vi "f_10_DiDtOff.vi"(0 "file path (IN)":path, 1 "Project #":string, 2 "Request #":string, 3 "TEST #":string, 5 "error in (no error)":errorcluster, 6 "ICE":dbl) -> (11 "Di (A)":dbl, 13 "Dt (ns)":dbl, 14 "file path (OUT)":path, 15 "Di/Dt (A/us)":dbl, 16 "DONE Di/Dt OFF":bool, 19 "error out":errorcluster)   [LabVIEW 2020]
uses:
  GlobIndSw1.vi
  <vilib>/Waveform/WDTOps.llb/WDT Waveform Duration DBL.vi
  <vilib>/Waveform/WDTOps.llb/WDT Get Waveform Subset DBL.vi
  <vilib>/measure/mamon.llb/Trigger Detection for 1 Channel.vi
  <vilib>/Analysis/NI_AALBase.lvlib
  <vilib>/measure/NI_MAPro.lvlib
panel:
  in  "Decision ?":bool
  out "Dt (us)":dbl
  out "50% Ice":dbl
  out "90% Ice":dbl
  out "Cursor a : Channel 1":dbl
  out "Cursor b : Channel 1":dbl
  out "Waveform Graph":waveform(dbl)[](graph)
  out "OFF Region":waveform(dbl)[](graph) caption="DiDtOff (A/us)"
  # "Di/dt(off): from 90% to 50% of the nominal current"
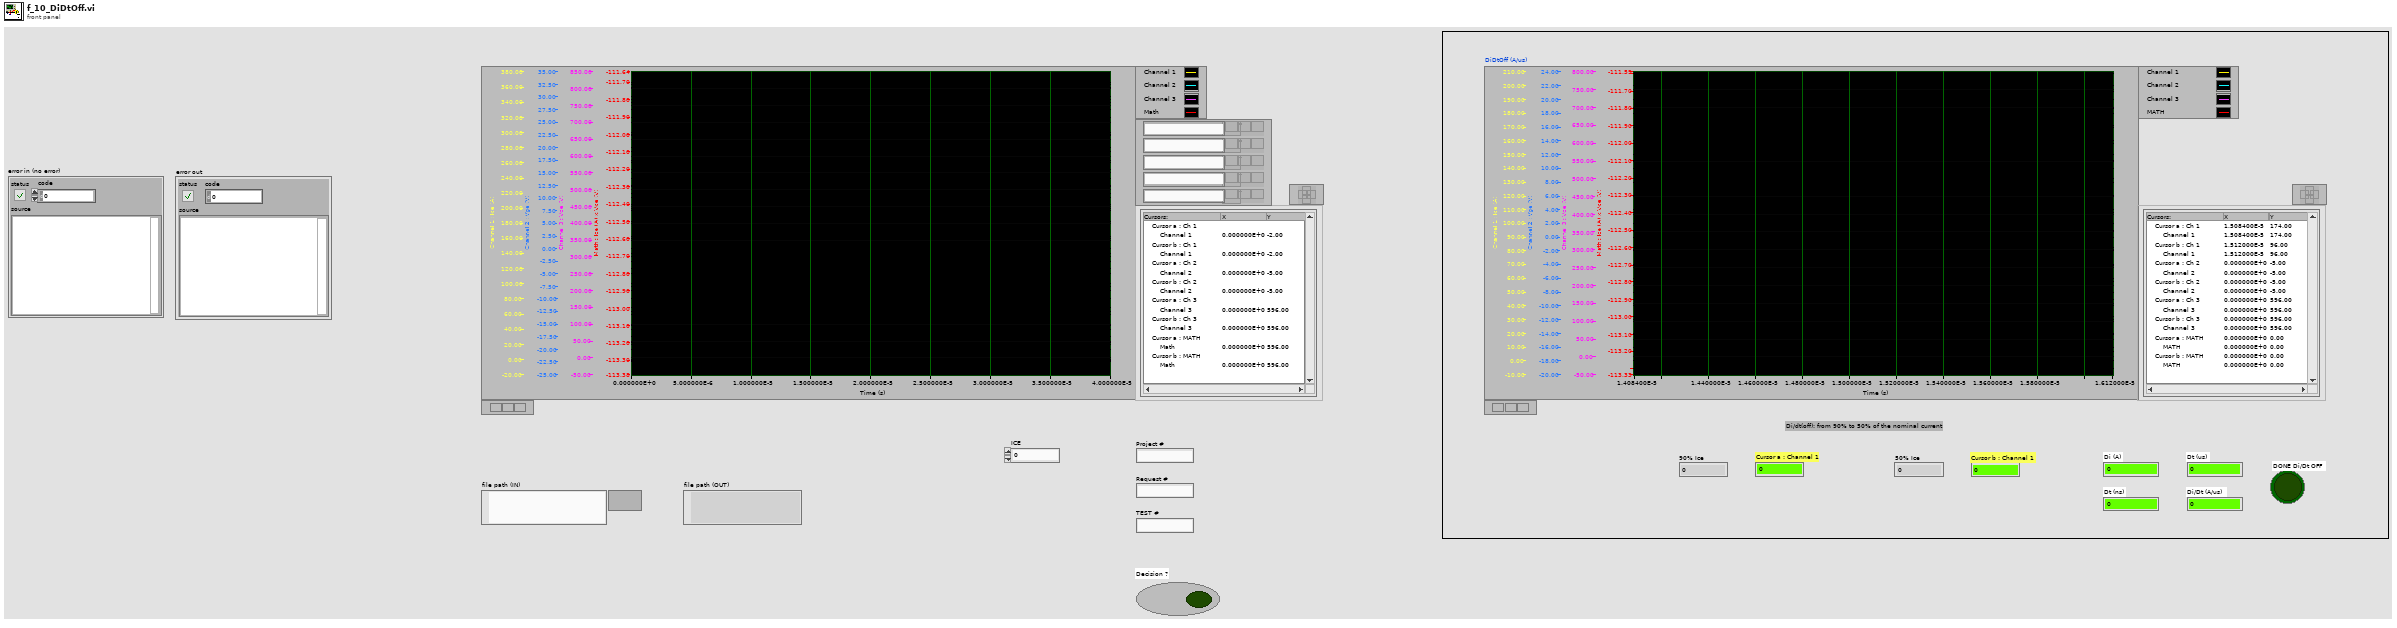
[diagram p1: front panel]
types:
  T1 = enum32{"Invalid", "Standard", "Closed", "Hidden", "Minimized", "Maximized"}
  T2 = typedef "imagedata.ctl" = cluster{"image type":i32, "image depth":i32, "image":u8[], "mask":u8[], "colors":u32[], "Rectangle":cluster{"left":i16, "top":i16, "right":i16, "bottom":i16}}
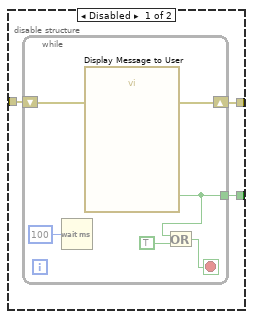
[diagram p3: hidden frame]
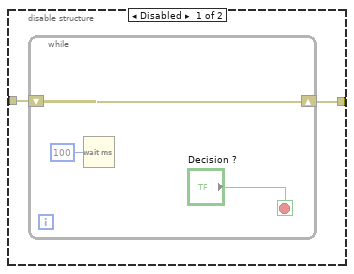
[diagram p8: hidden frame]
diagram:
  w2 = 0.0 ("Di (A)")
  w3 = errorcluster {"status"=FALSE, "code"=0, "source"=""} ("error out")
  w1 = FALSE ("DONE Tdon")
  w4 = waveform(dbl)[] [] ("Waveform Graph")
  n1 = disable-structure shown="Disabled" {
    frame Disabled {
      n2 = control-ref of="This VI"() -> (w11:refnum<vi>)
      n3 = control-ref of="This VI"() -> (w12:refnum<vi>)
      n4 = invoke class="VI" method="FP.Close"(reference=w11) -> ()  [unwired: 2 in, 3 out]
      n5 = invoke class="VI" method="FP.Open"(reference=w12, "Activate"=TRUE ("Activate?"), "State"=T1."Maximized") -> (error in=w15:errorcluster, error out=w13:errorcluster)  [unwired: 1 in, 4 out]
      n6 = property class="VI"(reference=w12, error in=w13, "Front Panel.Closeable"=TRUE ("Front Panel Window:Closeable")) -> ()  [unwired: 2 out]
    }
    frame Enabled {
    }
  }
  n7 = local write "Cursor a : Channel 1"(w2) -> ()
  n8 = local write "Cursor b : Channel 1"(w2) -> ()
  n9 = local write "Di (A)"(w2) -> ()
  n10 = local write "Dt (ns)"(w2) -> ()
  n11 = local write "Dt (us)"(w2) -> ()
  n12 = local write "Di/Dt (A/us)"(w2) -> ()
  n13 = local write "error out"(w3) -> ()
  n14 = local write "error in (no error)"(w3) -> ()
  n15 = local write "DONE Di/Dt OFF"(w1) -> ()
  n16 = local write "Waveform Graph"(w4) -> ()
  n17 = local write "OFF Region"(w4) -> ()
  n18 = local write "Decision ?"(w1) -> ()
  n19 = flat-sequence {
    tunnel: [w18] -> w10
    tunnel: ["file path (IN)"] -> w9
    tunnel: [w29] -> w8
    tunnel: [w28] -> w7
    tunnel: w10 -> [w27]
    tunnel: w9 -> [w26]
    tunnel: w8 -> [w287]
    tunnel: [w286] -> w6
    tunnel: w7 -> [w286]
    tunnel: [w285] -> w5
    tunnel: w6 -> [w301]
    tunnel: w5 -> [w300]
    frame #0 {
      n20 = control-ref of="This VI"() -> (w23:refnum<vi>)
      n21 = invoke class="VI" method="FP.Open"(reference=w23, error in="error in (no error)", "Activate"=TRUE ("Activate?"), "State"=T1."Maximized") -> (error out=w24:errorcluster)  [unwired: 1 in, 4 out]
      n22 = property class="VI"(reference=w23, error in=w24, "Front Panel.Closeable"=TRUE ("Front Panel Window:Closeable")) -> (error out=w18:errorcluster)  [unwired: 1 out]
    }
    frame #1 {
      n23 = while {
        tunnel: [w33] -> w28
        shift-right: [w34] -> w29
        shift-left: w27 -> [w32]
        tunnel: w26 -> [w31]
        stop <- w36 stop-if-true
        n24 = flat-sequence {
          tunnel: [w72] -> w55
          tunnel: w32 -> [w72]
          tunnel: w31 -> [w67]
          tunnel: [w67] -> w30
          tunnel: w55 -> [w169]
          tunnel: [w74] -> w54
          tunnel: [w94] -> w53
          tunnel: [w84] -> w52
          tunnel: w30 -> [w163]
          tunnel: w54 -> [w208]
          tunnel: w53 -> [w213]
          tunnel: [w224] -> w51
          tunnel: w52 -> [w233]
          tunnel: [w233] -> w50
          tunnel: [w221] -> w49
          tunnel: [w220] -> w48
          tunnel: [w205] -> w47
          tunnel: [w214] -> w46
          tunnel: w51 -> [w251]
          tunnel: [w252] -> w45
          tunnel: w50 -> [w255]
          tunnel: [w255] -> w44
          tunnel: w49 -> [w254]
          tunnel: [w254] -> w43
          tunnel: w48 -> [w253]
          tunnel: [w253] -> w42
          tunnel: w47 -> [w245]
          tunnel: [w245] -> w41
          tunnel: w46 -> [w246]
          tunnel: [w246] -> w40
          tunnel: w45 -> [w257]
          tunnel: w44 -> [w270]
          tunnel: [w270] -> w39
          tunnel: w43 -> [w264]
          tunnel: w42 -> [w265]
          tunnel: w41 -> [w263]
          tunnel: w40 -> [w262]
          tunnel: [w257] -> w38
          tunnel: w39 -> [w275]
          tunnel: w38 -> [w277]
          tunnel: [w276] -> w37
          tunnel: [w275] -> w33
          frame #0 {
            w70 = 0.0 ("Di (A)")
            w71 = FALSE ("DONE Tdon")
            w69 = waveform(dbl)[] [] ("Waveform Graph")
            n25 = Wait (ms)(milliseconds to wait=u32 400) -> ()  [unwired: 1 out]
            n26 = local write "Cursor a : Channel 1"(w70) -> ()
            n27 = local write "Cursor b : Channel 1"(w70) -> ()
            n28 = local write "Di/Dt (A/us)"(w70) -> ()
            n29 = local write "Dt (us)"(w70) -> ()
            n30 = local write "Di (A)"(w70) -> ()
            n31 = local write "Dt (ns)"(w70) -> ()
            n32 = local write "DONE Di/Dt OFF"(w71) -> ()
            n33 = local write "Waveform Graph"(w69) -> ()
            n34 = local write "OFF Region"(w69) -> ()
            n35 = local write "Decision ?"(w71) -> ()
          }
          frame #1 {
            w78 = 0.0 ("start samples/time")
            w144 = u16 1 items=["Samples", "Relative Time"] ("start/duration format")
            w155 = u16 1 items=["Samples", "Relative Time"] ("start/duration format")
            w156 = u16 1 items=["Samples", "Relative Time"] ("start/duration format")
            # "Channel 1"
            # "Channel 3"
            # "Channel 2"
            # "dt"
            # "Ch2"
            # "Ch1"
            n36 = call "3_ReadDatatoWaveform.vi"("error in (no error)"=w169, "file path (IN)"=w163) -> ("error out"=w77:errorcluster, "Waveform Graph"=→"Waveform Graph":waveform(dbl)[], "file path (OUT)"=w84:path, "dt"=w164:dbl, "Ch 2 Data"=w161:dbl[], "Ch 3 Data"=w165:dbl[], "Ch 1 Data"=w162:dbl[])  [unwired: 3 in]
            n37 = call <vilib>:"Beep.vi"("use system alert? (T)"=FALSE, "duration (msec)"=u32 200, "frequency (Hz)"=u32 2000) -> ()  [unwired: 9 in]
            n38 = Wait (ms)(milliseconds to wait=u32 400) -> ()  [unwired: 1 out]
            n39 = To Time Stamp(1:0.0 ("number")) -> (0:w166:timestamp)
            n40 = disable-structure shown="Enabled" {
              disable-tunnel: w166 -> [w197 _]
              disable-tunnel: w164 -> [w196 _]
              disable-tunnel: w165 -> [w195 _]
              disable-tunnel: [w194 _] -> w142
              frame Enabled {
                # "Channel 3"
                n41 = Bundle By Name("Y"=w195, "dt"=w196, "t0"=w197) -> (w194:waveform(dbl))  [unwired: 1 in]
              }
              frame Disabled {
              }
            }
            n42 = disable-structure shown="Enabled" {
              disable-tunnel: w166 -> [w189 _]
              disable-tunnel: w164 -> [w188 _]
              disable-tunnel: w162 -> [w187 _]
              disable-tunnel: [w186 _] -> w75
              frame Enabled {
                # "Channel 1"
                n43 = Bundle By Name("Y"=w187, "dt"=w188, "t0"=w189) -> (w186:waveform(dbl))  [unwired: 1 in]
              }
              frame Disabled {
              }
            }
            n44 = disable-structure shown="Enabled" {
              disable-tunnel: w166 -> [w193 _]
              disable-tunnel: w164 -> [w192 _]
              disable-tunnel: w161 -> [w191 _]
              disable-tunnel: [w190 _] -> w143
              frame Enabled {
                # "Channel 2"
                n45 = Bundle By Name("Y"=w191, "dt"=w192, "t0"=w193) -> (w190:waveform(dbl))  [unwired: 1 in]
              }
              frame Disabled {
              }
            }
            n46 = disable-structure shown="Enabled" {
              disable-tunnel: w75 -> [w182 _]
              disable-tunnel: w77 -> [w174 _]
              disable-tunnel: [w173 _] -> w76
              disable-tunnel: [w172 _] -> w74
              disable-tunnel: w78 -> [w171 _]
              frame Enabled {
                w176 = u16 1 items=["Samples", "Relative Time"] ("start/duration format")
                # "Channel 1 - Filtered"
                # "Median"
                n47 = global read "GlobIndSw1.vi" "Median Filter Rank"() -> (w170:i32)
                n48 = Unbundle By Name(w182) -> ("Y"=w185:dbl[], "dt"=w183:dbl)
                n49 = call <vilib>:"Median Filter.vi"("right rank"=w170, "left rank"=w170, "X"=w185) -> ("Filtered X"=w184:dbl[])  [unwired: 7 in, 1 out]
                n50 = Bundle By Name("Y"=w184, "dt"=w183) -> (w175:waveform(dbl))  [unwired: 1 in]
                n51 = call-poly <vilib>:"Waveform Duration.vi"("error in (no error)"=w174, "waveform in"=w175) -> ("error out"=w179:errorcluster, "duration"=w181:dbl, "waveform out"=w180:waveform(dbl))  [unwired: 7 in]
                n52 = Divide(x=w181, y=2.0) -> (x/y=w178:dbl)
                n53 = call-poly <vilib>:"Get Waveform Subset.vi"("start/duration format"=w176, "error in (no error)"=w179, "duration"=w178, "start samples/time"=w171, "waveform in"=w180) -> ("error out"=w173:errorcluster, "waveform out"=w172:waveform(dbl))  [unwired: 1 in, 2 out]
              }
              frame Disabled {
              }
            }
            n54 = call-poly <vilib>:"Waveform Duration.vi"("error in (no error)"=w77, "waveform in"=w142) -> ("error out"=w149:errorcluster, "duration"=w146:dbl, "waveform out"=w148:waveform(dbl))  [unwired: 7 in]
            n55 = call-poly <vilib>:"Waveform Duration.vi"("error in (no error)"=w77, "waveform in"=w143) -> ("error out"=w150:errorcluster, "duration"=w153:dbl, "waveform out"=w151:waveform(dbl))  [unwired: 7 in]
            n56 = call-poly <vilib>:"Waveform Duration.vi"("error in (no error)"=w77, "waveform in"=w75) -> ("error out"=w160:errorcluster, "duration"=w157:dbl, "waveform out"=w159:waveform(dbl))  [unwired: 7 in]
            n57 = Divide(x=w146, y=2.0) -> (x/y=w145:dbl)
            n58 = Divide(x=w153, y=2.0) -> (x/y=w154:dbl)
            n59 = Divide(x=w157, y=2.0) -> (x/y=w139:dbl)
            n60 = call-poly <vilib>:"Get Waveform Subset.vi"("start/duration format"=w144, "error in (no error)"=w149, "duration"=w145, "start samples/time"=w78, "waveform in"=w148) -> ("error out"=w80:errorcluster, "waveform out"=w141:waveform(dbl))  [unwired: 1 in, 2 out]
            n61 = call-poly <vilib>:"Get Waveform Subset.vi"("start/duration format"=w155, "error in (no error)"=w150, "duration"=w154, "start samples/time"=w78, "waveform in"=w151) -> ("error out"=w137:errorcluster, "waveform out"=w96:waveform(dbl))  [unwired: 1 in, 2 out]
            n62 = call-poly <vilib>:"Get Waveform Subset.vi"("start/duration format"=w156, "error in (no error)"=w160, "duration"=w139, "start samples/time"=w78, "waveform in"=w159) -> ("error out"=w138:errorcluster, "waveform out"=w95:waveform(dbl))  [unwired: 1 in, 2 out]
            n63 = Build Array(w95, w96, w141, waveform(dbl) {"t0"=timestamp(0 s since 1904-01-01), "dt"=1.0, "Y"=[]} ("element")) -> (→"OFF Region":waveform(dbl)[])
            n64 = Merge Errors(w138, w137, w80, w76) -> (w92:errorcluster)
            n65 = property on="OFF Region" class="WFGraph (strict)"(error in=w92) -> (error out=w91:errorcluster, "Width"=w90:u32)  [unwired: 1 in, 1 out]
            n66 = property on="OFF Region" class="WFGraph (strict)"(error in=w91, "Caption.Justify"=enum16{"Left", "Center", "Right"}."Left" ("Caption.Justification"), "Caption.Width"=w90, "Caption.FontBold"=TRUE ("Caption.Font:Bold"), "Caption.FontColor"=u32 16860 ("Caption.Font:Color"), "Caption.FontSize"=u32 24 ("Caption.Font:Size"), "Caption.Text"="DiDtOff (A/us)") -> (error out=w86:errorcluster)  [unwired: 1 in, 1 out]
            n67 = property on="OFF Region" class="WFGraph (strict)"(error in=w86, "XScale.Offset"=w78) -> (error out=w120:errorcluster)  [unwired: 1 in, 1 out]
            n68 = property on="OFF Region" class="WFGraph (strict)"(error in=w120, "Active Cursor"=u32 0, "Cursor.Cursor X"=0.0 ("Cursor.Cursor Position:Cursor X"), "Cursor.Cursor Y"=0.0 ("Cursor.Cursor Position:Cursor Y"), "Cursor.Visible"=FALSE) -> (error out=w119:errorcluster)  [unwired: 1 in, 1 out]
            n69 = property on="OFF Region" class="WFGraph (strict)"(error in=w119, "Active Cursor"=u32 1, "Cursor.Cursor X"=0.0 ("Cursor.Cursor Position:Cursor X"), "Cursor.Cursor Y"=0.0 ("Cursor.Cursor Position:Cursor Y"), "Cursor.Visible"=FALSE) -> (error out=w118:errorcluster)  [unwired: 1 in, 1 out]
            n70 = property on="OFF Region" class="WFGraph (strict)"(error in=w118, "Active Cursor"=u32 2, "Cursor.Cursor X"=0.0 ("Cursor.Cursor Position:Cursor X"), "Cursor.Cursor Y"=0.0 ("Cursor.Cursor Position:Cursor Y"), "Cursor.Visible"=FALSE) -> (error out=w117:errorcluster)  [unwired: 1 in, 1 out]
            n71 = property on="OFF Region" class="WFGraph (strict)"(error in=w117, "Active Cursor"=u32 3, "Cursor.Cursor X"=0.0 ("Cursor.Cursor Position:Cursor X"), "Cursor.Cursor Y"=0.0 ("Cursor.Cursor Position:Cursor Y"), "Cursor.Visible"=FALSE) -> (error out=w100:errorcluster)  [unwired: 1 in, 1 out]
            n72 = property on="OFF Region" class="WFGraph (strict)"(error in=w100, "Active Cursor"=u32 4, "Cursor.Cursor X"=0.0 ("Cursor.Cursor Position:Cursor X"), "Cursor.Cursor Y"=0.0 ("Cursor.Cursor Position:Cursor Y"), "Cursor.Visible"=FALSE) -> (error out=w99:errorcluster)  [unwired: 1 in, 1 out]
            n73 = property on="OFF Region" class="WFGraph (strict)"(error in=w99, "Active Cursor"=u32 5, "Cursor.Cursor X"=0.0 ("Cursor.Cursor Position:Cursor X"), "Cursor.Cursor Y"=0.0 ("Cursor.Cursor Position:Cursor Y"), "Cursor.Visible"=FALSE) -> (error out=w98:errorcluster)  [unwired: 1 in, 1 out]
            n74 = property on="OFF Region" class="WFGraph (strict)"(error in=w98, "Active Cursor"=u32 6, "Cursor.Cursor X"=0.0 ("Cursor.Cursor Position:Cursor X"), "Cursor.Cursor Y"=0.0 ("Cursor.Cursor Position:Cursor Y"), "Cursor.Visible"=FALSE) -> (error out=w97:errorcluster)  [unwired: 1 in, 1 out]
            n75 = property on="OFF Region" class="WFGraph (strict)"(error in=w97, "Active Cursor"=u32 7, "Cursor.Cursor X"=0.0 ("Cursor.Cursor Position:Cursor X"), "Cursor.Cursor Y"=0.0 ("Cursor.Cursor Position:Cursor Y"), "Cursor.Visible"=FALSE) -> (error out=w94:errorcluster)  [unwired: 1 in, 1 out]
          }
          frame #2 {
            w211 = u16 0 items=["Falling Edge", "Rising Edge"] ("trigger slope")
            w212 = u16 1 items=["Index", "Time"] ("location mode")
            w218 = u16 0 items=["Falling Edge", "Rising Edge"] ("trigger slope")
            w219 = u16 1 items=["Index", "Time"] ("location mode")
            # "XPOS"
            # "YPOS"
            # "Cursor a : Channel 1"
            # "Cursor b : Channel 1"
            # "Cursor b : Channel 1"
            # "Cursor a : Channel 1"
            # "Cursor b : Channel 1"
            # "Cursor a : Channel 1"
            # "Cursor b : Channel 1"
            # "Cursor a : Channel 1"
            # "End Time 1st Cursor"
            # "End Time 2nd Cursor"
            # "1st PARAMETER : 90% Ice"
            # "Channel 1"
            # "2nd PARAMETER : 50% Ice"
            # "Channel 1"
            n76 = Wait (ms)(milliseconds to wait=u32 500) -> ()  [unwired: 1 out]
            n77 = call <vilib>:"Beep.vi"("use system alert? (T)"=FALSE, "duration (msec)"=u32 200, "frequency (Hz)"=u32 2000) -> ()  [unwired: 9 in]
            n78 = Divide(x=90.0, y=100.0) -> (x/y=w243:dbl)
            n79 = Multiply(x=w243, y="ICE") -> (x*y=w215:dbl)
            "90% Ice" <- w215
            n80 = Add(x=w215, y=0.2) -> (x+y=w203:dbl)
            n81 = Divide(x=w203, y=10.0) -> (x/y=w202:dbl)
            n82 = call-poly <vilib>:"Basic Level Trigger Detection.vi"("signal in"=w208, "level"=w203, "hysteresis"=w202, "location mode"=w219, "error in (no error)"=w213, "trigger slope"=w218) -> ("trigger location"=w214:dbl, "error out"=w216:errorcluster)  [unwired: 7 in, 1 out]
            n83 = property on="OFF Region" class="WFGraph (strict)"(error in=w216, "Active Cursor"=u32 0, "Cursor.Cursor X"=w214, "Cursor.Visible"=TRUE, "Cursor.Cursor Name Visible"=TRUE) -> (error out=w228:errorcluster)  [unwired: 1 in, 1 out]
            n84 = property on="OFF Region" class="WFGraph (strict)"(error in=w228, "Active Cursor"=u32 0) -> (error out=w206:errorcluster, "Cursor.Cursor Y"=w221:dbl)  [unwired: 1 in, 1 out]
            "Cursor a : Channel 1" <- w221
            n85 = Divide(x=50.0, y=100.0) -> (x/y=w240:dbl)
            n86 = Multiply(x=w240, y="ICE") -> (x*y=w209:dbl)
            "50% Ice" <- w209
            n87 = Add(x=w209, y=0.2) -> (x+y=w200:dbl)
            n88 = Divide(x=w200, y=10.0) -> (x/y=w199:dbl)
            n89 = call-poly <vilib>:"Basic Level Trigger Detection.vi"("signal in"=w208, "level"=w200, "hysteresis"=w199, "location mode"=w212, "error in (no error)"=w206, "trigger slope"=w211) -> ("trigger location"=w205:dbl, "error out"=w207:errorcluster)  [unwired: 7 in, 1 out]
            n90 = property on="OFF Region" class="WFGraph (strict)"(error in=w207, "Active Cursor"=u32 1, "Cursor.Cursor X"=w205, "Cursor.Visible"=TRUE, "Cursor.Cursor Name Visible"=TRUE) -> (error out=w225:errorcluster)  [unwired: 1 in, 1 out]
            n91 = property on="OFF Region" class="WFGraph (strict)"(error in=w225, "Active Cursor"=u32 1) -> (error out=w224:errorcluster, "Cursor.Cursor Y"=w220:dbl)  [unwired: 1 in, 1 out]
            "Cursor b : Channel 1" <- w220
          }
          frame #3 {
            # "2nd Cursor"
            # "1st Cursor"
            n92 = Subtract(x=w246, y=1e-06) -> (x-y=w247:dbl)
            n93 = Add(x=w245, y=1e-06) -> (x+y=w248:dbl)
            n94 = property on="OFF Region" class="WFGraph (strict)"(error in=w251, "XScale.Minimum"=w247, "XScale.Maximum"=w248) -> (error out=w252:errorcluster)  [unwired: 1 in, 1 out]
            n95 = Wait (ms)(milliseconds to wait=u32 300) -> ()  [unwired: 1 out]
          }
          frame #4 {
            # "us"
            # "ns"
            n96 = Subtract(x=w265, y=w264) -> (x-y=w260:dbl)
            n97 = Subtract(x=w263, y=w262) -> (x-y=w261:dbl)
            n98 = Absolute Value(x=w260) -> (abs(x)=w259:dbl)
            "Di (A)" <- w259
            n99 = Absolute Value(x=w261) -> (abs(x)=w258:dbl)
            n100 = Multiply(x=w258, y=1000000000.0) -> (x*y=→"Dt (ns)":dbl)
            n101 = Multiply(x=w258, y=1000000.0) -> (x*y=w267:dbl)
            "Dt (us)" <- w267
            n102 = Wait (ms)(milliseconds to wait=u32 300) -> ()  [unwired: 1 out]
            n103 = call <vilib>:"Beep.vi"("use system alert? (T)"=FALSE, "duration (msec)"=u32 200, "frequency (Hz)"=u32 2000) -> ()  [unwired: 9 in]
            n104 = Divide(x=w259, y=w267) -> (x/y=→"Di/Dt (A/us)":dbl)
          }
          frame #5 {
            n105 = disable-structure shown="Enabled" {
              disable-tunnel: w277 -> [w279 w283]
              disable-tunnel: [w278 w283] -> w276
              frame Disabled {
                n106 = while {
                  shift-right: [w280] -> w278
                  shift-left: w279 -> [w280]
                  stop <- "Decision ?" stop-if-true
                  n107 = Wait (ms)(milliseconds to wait=u32 100) -> ()  [unwired: 1 out]
                }
              }
              frame Enabled {
              }
            }
          }
        }
        n108 = disable-structure shown="Enabled" {
          disable-tunnel: w37 -> [w58 w66]
          disable-tunnel: [w57 TRUE ("NO")] -> w36
          disable-tunnel: [w56 w66] -> w34
          frame Disabled {
            n109 = while {
              tunnel: [w60] -> w57
              shift-right: [w63] -> w56
              shift-left: w58 -> [w64]
              stop <- w62 stop-if-true
              n110 = Wait (ms)(milliseconds to wait=u32 100) -> ()  [unwired: 1 out]
              n111 = call "Display Message to User"("error in (no error)"=w64) -> ("error out"=w63:errorcluster, "NO"=w60:bool)  [unwired: 9 in]
              n112 = Or(x=w60, y=TRUE) -> (x .or. y?=w62:bool)
            }
          }
          frame Enabled {
          }
        }
        n113 = Wait (ms)(milliseconds to wait=u32 100) -> ()  [unwired: 1 out]
      }
    }
    frame #2 {
      w290 = "_"
      n114 = Wait (ms)(milliseconds to wait=u32 300) -> ()  [unwired: 1 out]
      n115 = invoke on="OFF Region" class="WFGraph (strict)" method="Get Image"(error in=w287) -> (error out=w293:errorcluster, "image data"=w296:T2)  [unwired: 5 in, 4 out]
      n116 = Concatenate Strings("C:\\Inductive_Switching_Project\\IndSw_Image\\" ("string"), "Project #", w290, "Request #", w290, "TEST #", w290, "DiDtOff" ("string"), ".png" ("string")) -> (w297:string)
      n117 = String To Path(string=w297) -> (path=w295:path)
      n118 = call <vilib>:"Write PNG File.vi"("error in (no error)"=w293, "image data"=w296, "path to PNG file"=w295) -> ("error out"=w285:errorcluster)  [unwired: 7 in, 1 out]
      "DONE Di/Dt OFF" <- TRUE ("DONE Di/Dt ON")
    }
    frame #3 {
      n119 = disable-structure shown="Enabled" {
        disable-tunnel: w300 -> [w302 _]
        frame Enabled {
          n120 = control-ref of="This VI"() -> (w303:refnum<vi>)
          n121 = invoke class="VI" method="FP.Close"(reference=w303, error in=w302) -> ()  [unwired: 1 in, 3 out]
        }
        frame Disabled {
        }
      }
      "error out" <- w300
      "file path (OUT)" <- w301
    }
  }
